vi "RSZVB Get TRM Measure Input.vi"(8 "error in (no error)":errorcluster {"code" format="%.0x"}, 9 "Path (1)":i32=1, 10 "Channel (1)":i32=1, 11 "VISA resource name":refnum<visa-resource-name>) -> (0 "error out":errorcluster {"code" format="%.0x"}, 2 "Input":i32, 3 "VISA resource name out":refnum<visa-resource-name>)   [LabVIEW 2011]
doc: "This VI returns the input for the a-wave (REF) receiver at paths no. 1-4.\n\nRemote-control command(s):\n[SENSe<Ch>:]TEUNit:AMONitor<Path>?"
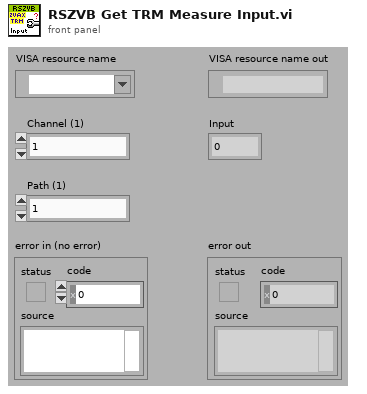
[diagram p1: front panel]
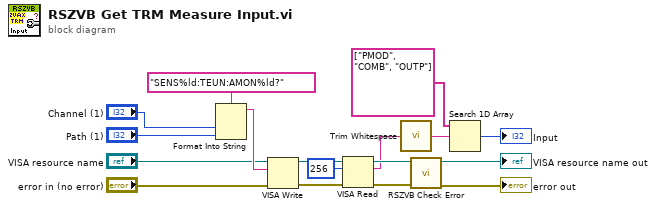
[diagram p0: block diagram]
diagram:
  n1 = Format Into String(format string="SENS%ld:TEUN:AMON%ld?", "Channel (1)", "Path (1)") -> (resulting string=w17:string)  [unwired: 2 in, 1 out]
  n2 = VISA Write(VISA resource name="VISA resource name", write buffer=w17, error in (no error)="error in (no error)") -> (VISA resource name out=w8:refnum<visa-resource-name>, error out=w7:errorcluster)  [unwired: 1 out]
  n3 = VISA Read(VISA resource name=w8, byte count=u32 256, error in (no error)=w7) -> (VISA resource name out=w5:refnum<visa-resource-name>, read buffer=w4:string, error out=w6:errorcluster)  [unwired: 1 out]
  n4 = call <vilib>:"Trim Whitespace.vi"("string"=w4) -> ("trimmed string"=w3:string)  [unwired: 1 in]
  n5 = call "RSZVB Check Error.vi"("error in (no error)"=w6, "VISA session"=w5) -> ("error out"=→"error out":errorcluster, "dup VISA session"=→"VISA resource name out":refnum<visa-resource-name>)  [unwired: 8 in]
  n6 = Search 1D Array(1D array=string[] ["PMOD", "COMB", "OUTP"], element=w3) -> (index of element=→"Input":i32)  [unwired: 1 in]
